vi "TC_GetStrFromRefArray.vi"(5 "arrayIn":T1, 10 "index":i32, 11 "NameToFind":string) -> (0 "arrayOut":T1, 3 "value":string)   [LabVIEW 2017]
uses:
  RefArray.ctl
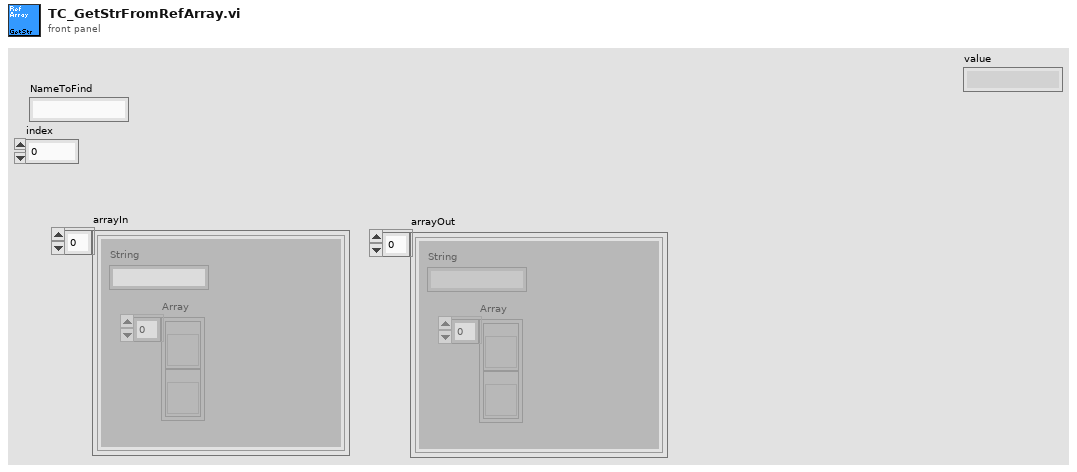
[diagram p1: front panel]
types:
  T1 = typedef "RefArray.ctl" = cluster{"String":string, "Array":refnum<vi>[]}[]
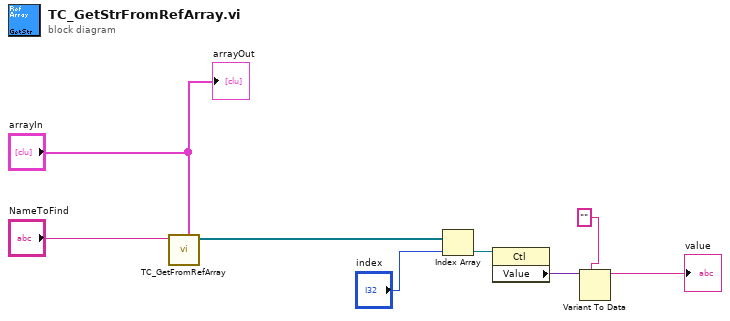
[diagram p0: block diagram]
diagram:
  n1 = call "TC_GetFromRefArray.vi"("arrayIn"="arrayIn", "NameToFind"="NameToFind") -> ("refArray"=w1:refnum<vi>[])  [unwired: 8 in, 1 out]
  n2 = Index Array(array=w1, index="index") -> (element=w7:refnum<vi>)
  n3 = property class="Ctl"(reference=w7) -> ("Value"=w8:variant)  [unwired: 1 in, 2 out]
  n4 = Variant To Data(type="", Variant=w8) -> (data=→"value":string)  [unwired: 1 in, 1 out]
  "arrayOut" <- "arrayIn"
